vi "Czytam6221_z_bufora_Wszystkie_POM_2008.vi"(4 "?":refnum<visa-resource-name>="GPIB0::6::INSTR") -> (3 "?":refnum<visa-resource-name>)   [LabVIEW 2012]
panel:
  out "Path Out":path
  out "output file 1:":path
  out "concatenated string":string
  out "decimal integer string":string
  out "read buffer 2":string
  in  "write buffer2":string="Trace:points:actual?"
  in  "write buffer 1":string="format:elements Reading, Source, AVOLTAGE"
  out "read buffer":string
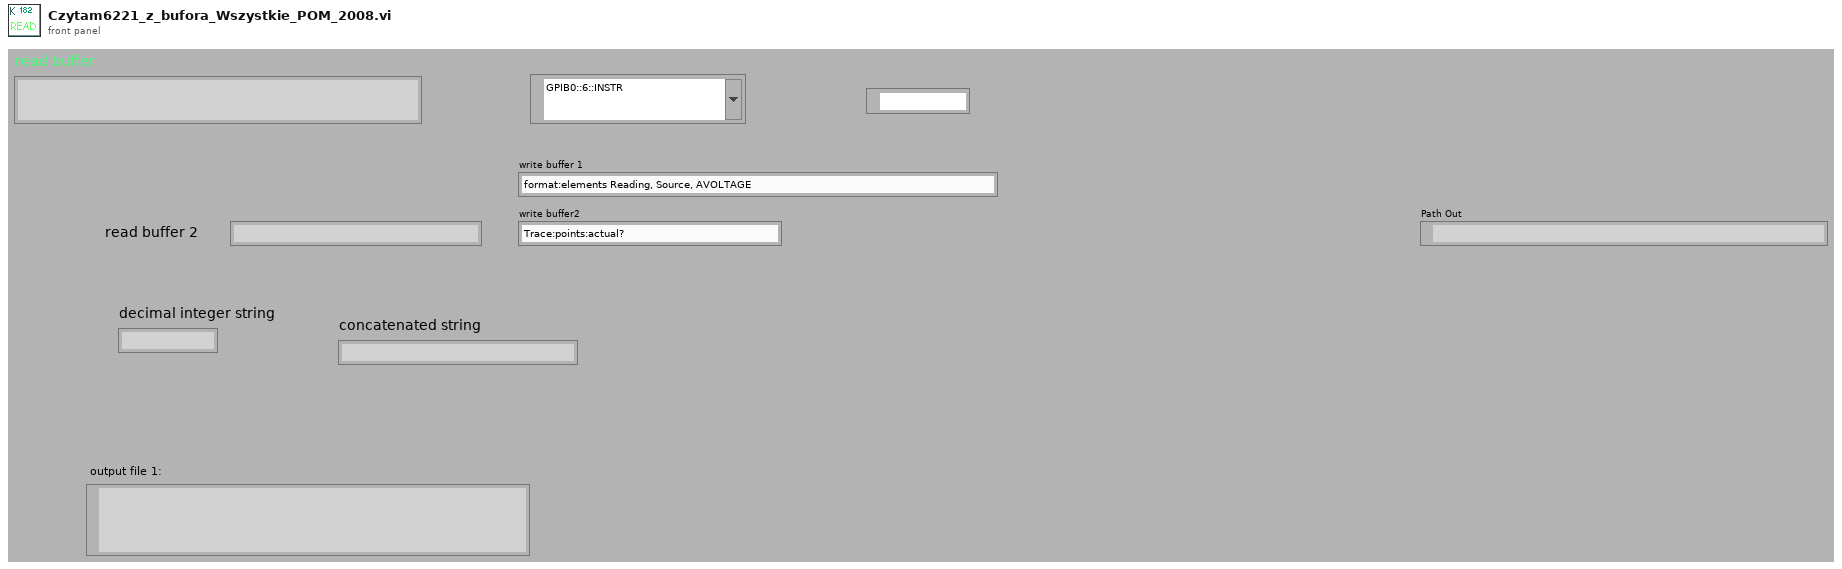
[diagram p1: front panel]
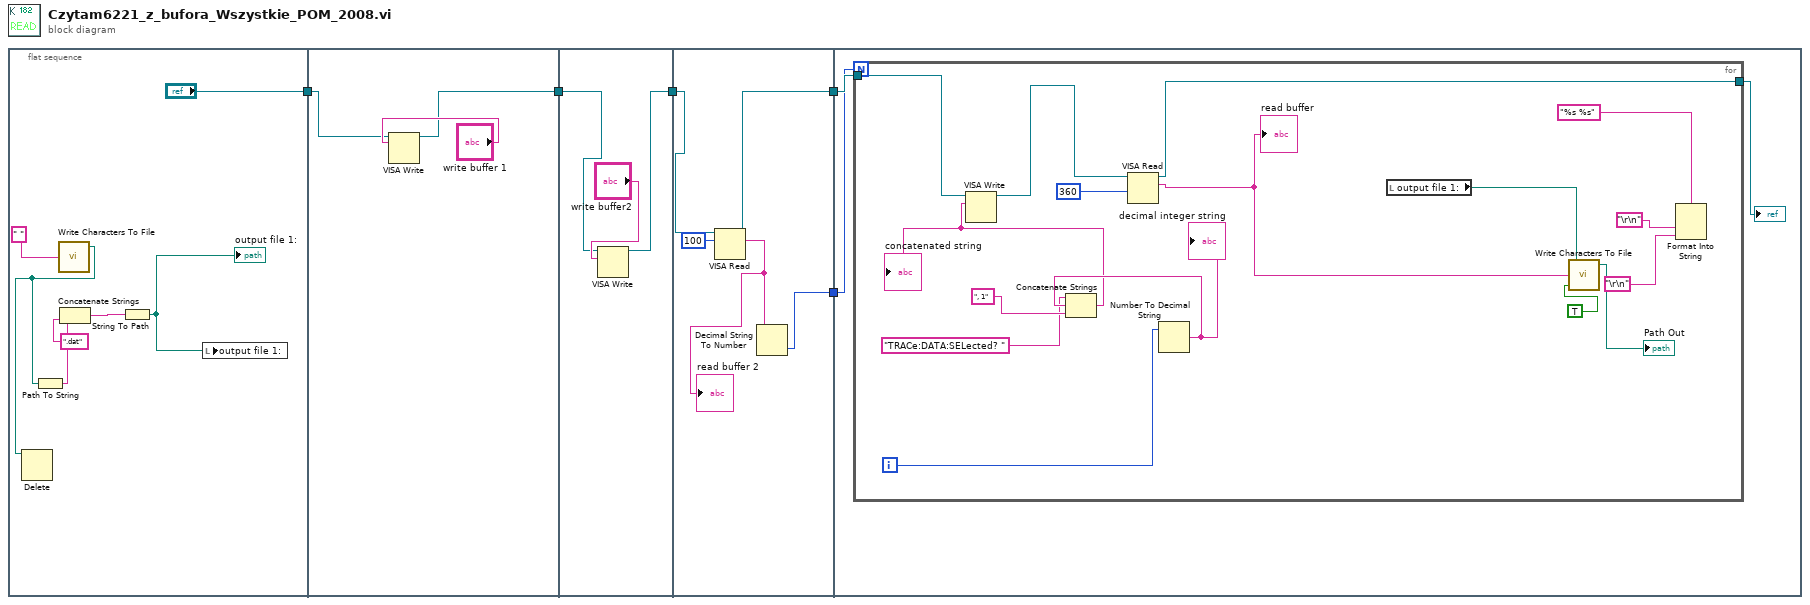
[diagram p0: block diagram]
diagram:
  n1 = flat-sequence {
    tunnel: ["?"] -> w5
    tunnel: w5 -> [w14]
    tunnel: [w13] -> w4
    tunnel: w4 -> [w17]
    tunnel: [w16] -> w3
    tunnel: w3 -> [w23]
    tunnel: [w22] -> w2
    tunnel: [w20] -> w1
    tunnel: w2 -> [w25]
    tunnel: w1 -> [w24]
    frame #0 {
      n2 = call <vilib>:"Write Characters To File.vi"("character string"=" ") -> ("new file path (Not A Path if cancelled)"=w6:path)  [unwired: 4 in]
      n3 = Delete(path (use dialog)=w6) -> ()  [unwired: 4 in, 3 out]
      n4 = Path To String(path=w6) -> (string=w9:string)
      n5 = Concatenate Strings(w9, ".dat") -> (w10:string)
      n6 = String To Path(string=w10) -> (path=w7:path)
      "output file 1:" <- w7
      n7 = local write "output file 1:"(w7) -> ()
    }
    frame #1 {
      n8 = VISA Write(VISA resource name=w14, write buffer="write buffer 1") -> (VISA resource name out=w13:refnum<visa-resource-name>)  [unwired: 1 in, 2 out]
    }
    frame #2 {
      n9 = VISA Write(VISA resource name=w17, write buffer="write buffer2") -> (VISA resource name out=w16:refnum<visa-resource-name>)  [unwired: 1 in, 2 out]
    }
    frame #3 {
      n10 = VISA Read(VISA resource name=w23, byte count=u32 100) -> (VISA resource name out=w22:refnum<visa-resource-name>, read buffer=w19:string)  [unwired: 1 in, 2 out]
      "read buffer 2" <- w19
      n11 = Decimal String To Number(string=w19) -> (number=w20:i32)  [unwired: 2 in, 1 out]
    }
    frame #4 {
      n12 = for {
        N: w24 -> [_]
        tunnel: [w42] -> w26
        tunnel: w25 -> [w41]
        i -> [w38]
        n13 = Number To Decimal String(number=w38) -> (decimal integer string=w37:string)  [unwired: 1 in]
        "decimal integer string" <- w37
        n14 = Concatenate Strings("TRACe:DATA:SELected? " ("write buffer"), w37, ", 1" ("write buffer")) -> (w36:string)
        "concatenated string" <- w36
        n15 = VISA Write(VISA resource name=w41, write buffer=w36) -> (VISA resource name out=w39:refnum<visa-resource-name>)  [unwired: 1 in, 2 out]
        n16 = VISA Read(VISA resource name=w39, byte count=u32 360) -> (VISA resource name out=w42:refnum<visa-resource-name>, read buffer=w28:string)  [unwired: 1 in, 2 out]
        "read buffer" <- w28
        n17 = local read "output file 1:"() -> (w31:path)
        n18 = call <vilib>:"Write Characters To File.vi"("append to file? (new file:F)"=TRUE, "character string"=w28, "file path (dialog if empty)"=w31) -> ("new file path (Not A Path if cancelled)"=→"Path Out":path)  [unwired: 2 in]
        n19 = Format Into String(format string="%s %s", "\r\n", "\r\n") -> ()  [unwired: 2 in, 2 out]
      }
      "?" <- w26
    }
  }
